vi "channel add.vi"(10 "number of channels (1)":i32=1) -> (0 "error out":errorcluster, 1 "lines match?":bool, 2 "channels":refnum<class "TBM channel.lvclass">[](array[class]), 3 "configuration out":refnum<class "shared memory configuration.lvclass">, 4 "valid?":bool)   [LabVIEW 2013, in "shared memory tests.lvlib"]
uses:
  shared memory tests.lvlib
  <vilib>/NI/Configuration Framework/serializable configuration/NISE_CEF_serializable configuration.lvclass
  module/configuration/shared memory configuration.lvclass
  <vilib>/NI/Tag Bus/tag/tag descriptor.lvclass
  <vilib>/NI/Tag Bus/tag/Data Type.ctl
  <vilib>/NI/Tag Bus Module Framework/channel/TBM channel.lvclass
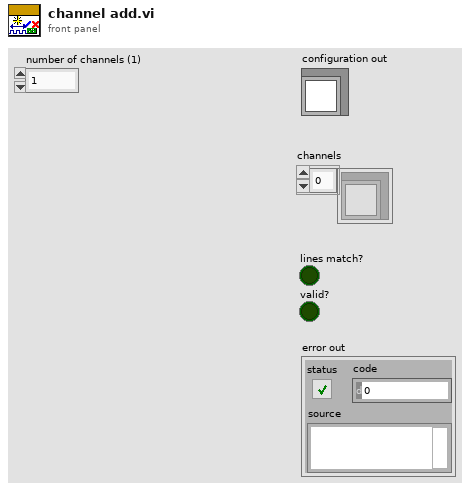
[diagram p1: front panel]
types:
  T1 = typedef "tag bus.lvlib/tag descriptor.lvclass/Data Type.ctl" = enum16{"Double", "Single", "I64", "I32", "I16", "I8", "U64", "U32", "U16", "U8", "Boolean", "String", "Array of Double", "Array of Single", "Array of I64", "Array of I32", "Array of I16", "Array of I8", "Array of U64", "Array of U32", "Array of U16", "Array of U8", "Array of Boolean", "Array of String"}
  T2 = typedef "TBM channel.lvclass/channel classification.ctl" = enum16{"input data", "output data", "processing parameter", "processing result"}
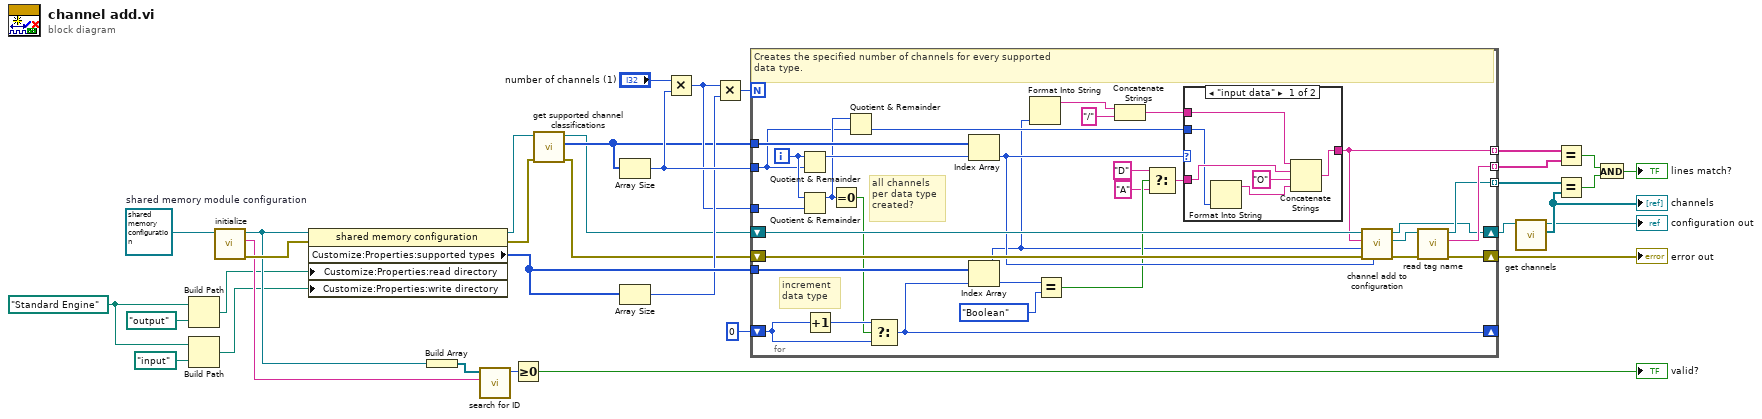
[diagram p0: block diagram]
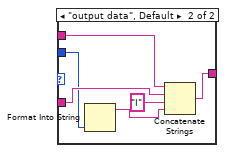
[diagram p2: hidden frame]
diagram:
  w6 = path "Standard Engine"
  w33 = refnum<class "shared memory configuration.lvclass"> refnum  # shared memory module configuration
  n1 = Build Path(base path=w6, name or relative path=path "output") -> (appended path=w16:path)
  n2 = Build Path(base path=w6, name or relative path=path "input") -> (appended path=w15:path)
  n3 = call <vilib>:"initialize.vi"("configuration in"=w33) -> ("error out"=w34:errorcluster, "identifier"=w25:string, "configuration out"=w27:refnum<class "shared memory configuration.lvclass">)  [unwired: 8 in]
  n4 = property class="shared memory configuration"(reference=w27, error in=w34, "Customize:Properties:read directory"=w16, "Customize:Properties:write directory"=w15) -> (reference out=w2:refnum<class "shared memory configuration.lvclass">, error out=w4:errorcluster, "Customize:Properties:supported types"=w14:T1[])
  n5 = Build Array(w27) -> (w26:refnum<class "shared memory configuration.lvclass">[])
  n6 = call <vilib>:"search for ID.vi"("instance id"=w25, "instance data"=w26) -> ("index"=w24:i32)  [unwired: 9 in]
  n7 = Greater Or Equal To 0?(x=w24) -> (x >= 0?=→"valid?":bool)
  n8 = call-dynamic "get supported channel classifications.vi"("error in"=w4, "module configuration in"=w2) -> ("error out"=w3:errorcluster, "supported types"=w5:T2[], "module configuration out"=w1:refnum<class "shared memory configuration.lvclass">)  [unwired: 7 in]
  n9 = Array Size(array=w5) -> (size(s)=w10:i32)
  n10 = Array Size(array=w14) -> (size(s)=w9:i32)
  n11 = Multiply(x="number of channels (1)", y=w10) -> (x*y=w7:i32)
  n12 = Multiply(x=w7, y=w9) -> (x*y=w8:i32)
  n13 = for {
    N: w8 -> [_]
    shift-right: [w58] -> w32
    shift-left: w1 -> [w64]
    shift-right: [w59] -> w13
    shift-left: w3 -> [w65]
    tunnel: w14 -> [w56]
    tunnel: [w60] -> w29 mode=indexing
    tunnel: [w61] -> w30 mode=indexing
    tunnel: [w57] -> w31 mode=indexing
    tunnel: w5 -> [w55]
    tunnel: w10 -> [w40]
    shift-right: [w44] -> _
    shift-left: 0 -> [w51]
    tunnel: w7 -> [w52]
    i -> [w53]
    # "increment \ndata type"
    # "all channels \nper data type \ncreated?"
    # "Creates the specified number of channels for every supported\ndata type."
    n14 = Quotient & Remainder(x=w53, y=w40) -> (x-y*floor(x/y)=w42:i32)  [unwired: 1 out]
    n15 = Quotient & Remainder(x=w53, y=w52) -> (x-y*floor(x/y)=w41:i32)  [unwired: 1 out]
    n16 = Increment(x=w51) -> (x+1=w50:i32)
    n17 = Equal To 0?(x=w41) -> (x = 0?=w43:bool)
    n18 = Quotient & Remainder(x=w41, y=w40) -> (floor(x/y)=w39:i32)  [unwired: 1 out]
    n19 = Select(t=w50, s=w43, f=w51) -> (s? t:f=w44:i32)
    n20 = Index Array(array=w55, index=w42) -> (element=w54:T2)
    n21 = Index Array(array=w56, index=w44) -> (element=w38:T1)
    n22 = Format Into String(w38) -> (resulting string=w37:string)  [unwired: 3 in, 1 out]
    n23 = Equal?(x=w38, y=Data_Type."Boolean" ("Data Type")) -> (x = y?=w48:bool)
    n24 = Concatenate Strings(w37, "/" ("string")) -> (w35:string)
    n25 = Select(t="D", s=w48, f="A") -> (s? t:f=w45:string)
    n26 = case shown="\"input data\"" w54 {
      tunnel: [w69 w75] -> w57
      tunnel: w45 -> [w68 w74]
      tunnel: w39 -> [w67 w73]
      tunnel: w35 -> [w66 w72]
      frame "input data" {
        n27 = Format Into String(w67) -> (resulting string=w70:string)  [unwired: 3 in, 1 out]
        n28 = Concatenate Strings(w66, w68, "O", w70) -> (w69:string)
      }
      frame "output data", Default {
        n29 = Format Into String(w73) -> (resulting string=w76:string)  [unwired: 3 in, 1 out]
        n30 = Concatenate Strings(w72, w74, "I", w76) -> (w75:string)
      }
    }
    n31 = call "channel add to configuration.vi"("channel classification (output data)"=w54, "error in"=w65, "data type"=w38, "channel name"=w57, "shared memory module configuration in"=w64) -> ("error out"=w62:errorcluster, "created channel"=w63:refnum<class "TBM channel.lvclass">, "shared memory module configuration out"=w58:refnum<class "shared memory configuration.lvclass">)  [unwired: 4 in]
    n32 = call <vilib>:"read tag name.vi"("error in"=w62, "system tag in"=w63) -> ("error out"=w59:errorcluster, "name"=w61:string, "system tag out"=w60:refnum<class "TBM channel.lvclass">)  [unwired: 7 in]
  }
  "error out" <- w13
  n33 = call-dynamic "get channels.vi"("shared memory configuration in"=w32) -> ("channels"=w28:refnum<class "TBM channel.lvclass">[], "shared memory configuration out"=→"configuration out":refnum<class "shared memory configuration.lvclass">)  [unwired: 9 in]
  "channels" <- w28
  n34 = Equal?(x=w31, y=w30) -> (x = y?=w21:bool)
  n35 = Equal?(x=w29, y=w28) -> (x = y?=w20:bool)
  n36 = And(x=w21, y=w20) -> (x .and. y?=→"lines match?":bool)
